vi "Create Unique Notifier ID.vi"(1 "Message Name":string) -> (0 "ID Out":string)   [LabVIEW 2019, in "Architecture.lvlib"]
doc: "This method generates a Unique ID to be used as the name of a notifier."
uses:
  Architecture.lvlib
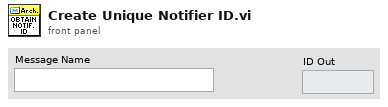
[diagram p1: front panel]
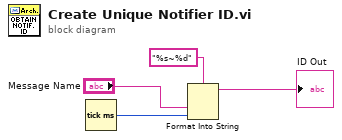
[diagram p0: block diagram]
diagram:
  n1 = Tick Count (ms)() -> (millisecond timer value=w2:u32)
  n2 = Format Into String(format string="%s~%d", "Message Name", w2) -> (resulting string=→"ID Out":string)  [unwired: 2 in, 1 out]
